vi "Test VI DD Functionality.vi"   [LabVIEW 2020]
uses:
  Oscilloscope.lvclass
  Oscilloscope VI/Oscilloscope VI.lvlib
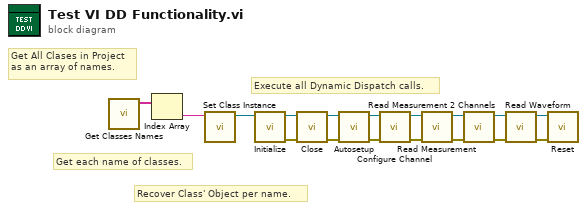
[diagram p0: block diagram]
diagram:
  # "Execute all Dynamic Dispatch calls."
  # "Recover Class' Object per name."
  # "Get each name of classes."
  # "Get All Clases in Project\nas an array of names."
  n1 = call "Get Classes Names.vi"() -> ("Classes Names"=w17:string[])  [unwired: 10 in, 1 out]
  n2 = Index Array(array=w17) -> (element=w2:string)  [unwired: 1 in]
  n3 = call "Set Class Instance.vi"("Oscilloscope Model"=w2) -> ("Oscilloscope"=w1:refnum<class "Oscilloscope.lvclass">)  [unwired: 9 in, 1 out]
  n4 = call-dynamic "Initialize.vi"("Oscilloscope in"=w1) -> ("error out"=w15:errorcluster, "Oscilloscope out"=w16:refnum<class "Oscilloscope.lvclass">)  [unwired: 9 in]
  n5 = call-dynamic "Close.vi"("error in (no error)"=w15, "Oscilloscope in"=w16) -> ("error out"=w13:errorcluster, "Oscilloscope out"=w14:refnum<class "Oscilloscope.lvclass">)  [unwired: 8 in]
  n6 = call-dynamic "Autosetup.vi"("error in (no error)"=w13, "Oscilloscope in"=w14) -> ("error out"=w11:errorcluster, "Oscilloscope out"=w12:refnum<class "Oscilloscope.lvclass">)  [unwired: 8 in]
  n7 = call-dynamic "Configure Channel.vi"("error in (no error)"=w11, "Oscilloscope in"=w12) -> ("error out"=w9:errorcluster, "Oscilloscope out"=w10:refnum<class "Oscilloscope.lvclass">)  [unwired: 8 in]
  n8 = call-dynamic "Read Measurement.vi"("error in (no error)"=w9, "Oscilloscope in"=w10) -> ("error out"=w7:errorcluster, "Oscilloscope out"=w8:refnum<class "Oscilloscope.lvclass">)  [unwired: 8 in]
  n9 = call-dynamic "Read Measurement 2 Channels.vi"("error in (no error)"=w7, "Oscilloscope in"=w8) -> ("error out"=w5:errorcluster, "Oscilloscope out"=w6:refnum<class "Oscilloscope.lvclass">)  [unwired: 8 in]
  n10 = call-dynamic "Read Waveform.vi"("error in (no error)"=w5, "Oscilloscope in"=w6) -> ("error out"=w3:errorcluster, "Oscilloscope out"=w4:refnum<class "Oscilloscope.lvclass">)  [unwired: 8 in]
  n11 = call-dynamic "Reset.vi"("error in (no error)"=w3, "Oscilloscope in"=w4) -> ()  [unwired: 8 in, 2 out]
